vi "GyroInit.vi"(0 "refnum name":string, 1 "Analog Channel":T1) -> ()   [LabVIEW 2011]
uses:
  <vilib>/Rock Robotics/SystemInterfaces/AI/FPGA_AIGyroChannel.ctl
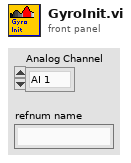
[diagram p1: front panel]
types:
  T1 = typedef "FPGA_AIGyroChannel.ctl" = enum8{"AI 1", "AI 2", "Invalid"}
  T2 = typedef "WPI_GyroDevRef.ctl" = cluster{"DevStatus":errorcluster, "Analog Module":T3, "Analog Channel":T4, "Offset":dbl, "Gain (VoltsPerDegree/Second)":dbl}
  T3 = typedef "FPGA_TypedefAnalogModule.ctl" = enum16{"Analog Module 1", "Analog Module 2"}
  T4 = typedef "FPGA_AIChannel.ctl" = enum8{"AI 1", "AI 2", "AI 3", "AI 4", "AI 5", "AI 6", "AI 7", "AI 8", "Invalid"}
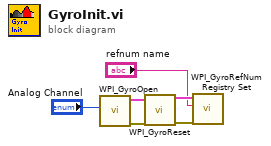
[diagram p0: block diagram]
diagram:
  n1 = call <vilib>:"WPI_GyroOpen.vi"("Analog Channel"="Analog Channel") -> ("error out"=w4:errorcluster, "GyroDevRef"=w3:T2)  [unwired: 8 in, 1 out]
  n2 = call <vilib>:"WPI_GyroReset.vi"("error in (no error)"=w4, "GyroDevRef"=w3) -> ("error out"=w5:errorcluster, "GyroDevRef"=w6:T2)  [unwired: 8 in]
  n3 = call <vilib>:"WPI_GyroRefNum Registry Set.vi"("error in (no error)"=w5, "refnum name"="refnum name", "GyroDevRef"=w6) -> ()  [unwired: 7 in, 2 out]
